vi "cDAQ Initialize.vi"(0 "DAQmx Task (Temperature)":refnum<k21>="Temperature", 1 "DAQmx Task (Analog Input Volt)":refnum<k21>="Temperature", 3 "Error In":errorcluster) -> (7 "Temp Task Out":refnum<k21>, 8 "AI Task Out":refnum<k21>, 10 "Error Out":errorcluster)   [LabVIEW 2014]
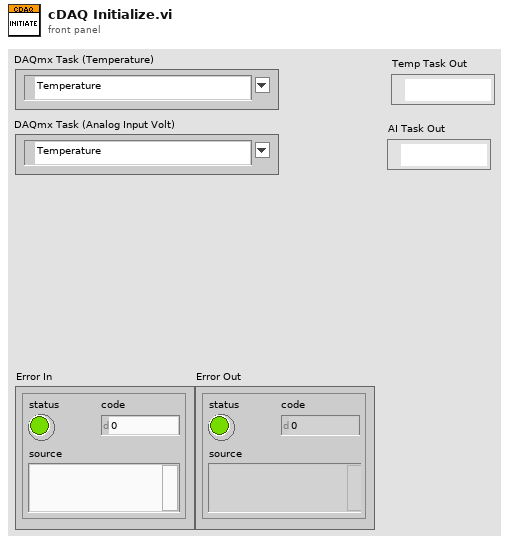
[diagram p1: front panel]
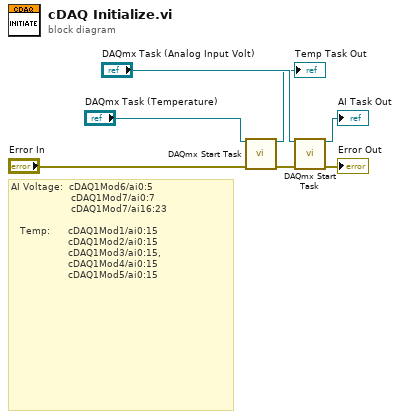
[diagram p0: block diagram]
diagram:
  # "AI Voltage:  cDAQ1Mod6/ai0:5\n                    cDAQ1Mod7/ai0:7\n                    cDAQ1Mod7/ai16:23\n\n   Temp:      cDAQ1Mod1/ai0:15\n                   cDAQ1Mod2/ai0:15\n                   cDAQ1Mod3/ai0:15,\n                   cDAQ1Mod4/ai0:15\n                   cDAQ1Mod5/ai0:15"
  n1 = call <vilib>:"DAQmx Start Task.vi"("task/channels in"="DAQmx Task (Temperature)", "error in"="Error In") -> ("task out"=→"Temp Task Out":refnum<k21>, "error out"=w5:errorcluster)  [unwired: 12 in]
  n2 = call <vilib>:"DAQmx Start Task.vi"("task/channels in"="DAQmx Task (Analog Input Volt)", "error in"=w5) -> ("task out"=→"AI Task Out":refnum<k21>, "error out"=→"Error Out":errorcluster)  [unwired: 12 in]
